vi "Initialize Logging.vi"(8 "error in (no error)":errorcluster, 11 "logging configuration":T1) -> (0 "error out":errorcluster, 3 "Producer":refnum<class "Word Log Producer.lvclass">)   [LabVIEW 2020, in "Ballard ARINC 429 Engine.lvlib" / "Custom Device.lvlib"]
uses:
  Custom Device.lvlib
  Logging Configuration.ctl
  Shared/Data Word Format.ctl
  Implementation/Logging/Word Log Producer/Word Log Producer.lvclass
  C:/Program Files (x86)/National Instruments/LabVIEW 2020/vi.lib/NI/VeriStand Custom Device Messaging/Producer/Abstract Producer/Abstract Producer.lvclass
  Implementation/Logging/CSV Word Logger/CSV Word Logger.lvclass
  C:/Git/niveristand-ballard-arinc429-custom-device/Source/Custom Device Support/Engine/Implementation/Logging/Word Logger Interface/Word Logger Interface.lvclass
  <vilib>/NI/VeriStand Custom Device Messaging/Message Queue/Message Queue/Message Queue.lvclass
  C:/Program Files (x86)/National Instruments/LabVIEW 2020/vi.lib/NI/VeriStand Custom Device Messaging/Message Queue/Abstract Message Queue/Abstract Message Queue.lvclass
  <vilib>/string/Create NI GUID.vi
  <vilib>/NI/VeriStand Custom Device Messaging/Consumer/Abstract Consumer/Initialize.vi
  <vilib>/NI/VeriStand Custom Device Messaging/Producer/Abstract Producer/Initialize.vi
  Implementation/Logging/Launch Message Handler.vi
  <vilib>/NI/VeriStand Custom Device Messaging/Consumer/Abstract Consumer/Abstract Consumer.lvclass
  <vilib>/NI/VeriStand Custom Device Messaging/Parameters/Abstract Init Parameters/Abstract Init Parameters.lvclass
  Implementation/Logging/Word Logging.lvlib
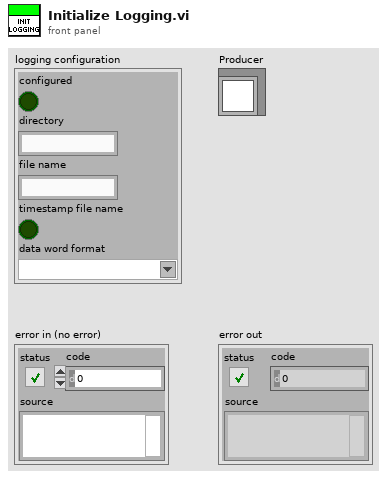
[diagram p1: front panel]
types:
  T1 = typedef "Ballard ARINC 429 Engine.lvlib/Custom Device.lvlib/Logging Configuration.ctl" = cluster{"configured":bool, "directory":string, "file name":string, "timestamp file name":bool, "data word format":T2}
  T2 = typedef "Data Word Format.ctl" = string
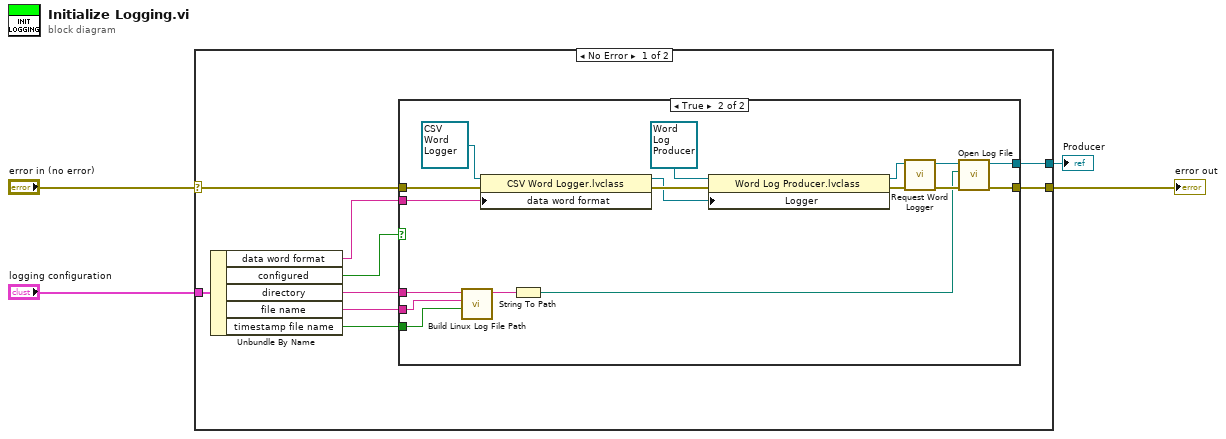
[diagram p0: block diagram]
diagram:
  n1 = case shown="No Error" "error in (no error)" {
    selector: "error in (no error)" -> [w13 w32]
    tunnel: "logging configuration" -> [w11 _]
    tunnel: [w10 w32] -> w2
    tunnel: [w9 _] -> w1
    frame No Error {
      n2 = Unbundle By Name(w11) -> ("data word format"=w7:T2, "configured"=w8:bool, "directory"=w12:string, "file name"=w6:string, "timestamp file name"=w5:bool)
      n3 = case shown="True" w8 {
        tunnel: w13 -> [w14 w28]
        tunnel: [w14 w26] -> w10
        tunnel: [_ w24] -> w9
        tunnel: w12 -> [_ w19]
        tunnel: w7 -> [_ w21]
        tunnel: w6 -> [_ w18]
        tunnel: w5 -> [_ w17]
        frame False {
        }
        frame True {
          n4 = call "Build Linux Log File Path.vi"("Timestamp"=w17, "Name"=w18, "Log File Directory"=w19) -> ("Log File Path"=w16:string)  [unwired: 7 in, 1 out]
          n5 = property class="CSV Word Logger.lvclass"(reference=refnum<class "CSV Word Logger.lvclass"> refnum ("Communication Bus Template Interfaces:Implementation.lvlib:Logging.lvlib:CSV Word Logger.lvclass"), error in=w28, "data word format"=w21) -> (reference out=w20:refnum<class "CSV Word Logger.lvclass">, error out=w23:errorcluster)
          n6 = String To Path(string=w16) -> (path=w15:path)
          n7 = property class="Word Log Producer.lvclass"(reference=refnum<class "Word Log Producer.lvclass"> refnum ("Communication Bus Template Interfaces:Implementation.lvlib:Logging.lvlib:Word Log Producer.lvclass"), error in=w23, "Logger"=w20) -> (reference out=w29:refnum<class "Word Log Producer.lvclass">, error out=w27:errorcluster)
          n8 = call "Request Word Logger.vi"("error in (no error)"=w27, "Producer in"=w29) -> ("error out"=w31:errorcluster, "Producer out"=w25:refnum<class "Word Log Producer.lvclass">)  [unwired: 8 in]
          n9 = call "Open Log File.vi"("error in (no error)"=w31, "Path"=w15, "Word Log Producer in"=w25) -> ("error out"=w26:errorcluster, "Word Log Producer out"=w24:refnum<class "Word Log Producer.lvclass">)  [unwired: 7 in]
        }
      }
    }
    frame Error {
    }
  }
  "error out" <- w2
  "Producer" <- w1
